vi "Increment.vi"(11 "Data Generator Actor in":refnum<class "Data Generator Actor.lvclass">) -> (3 "Data Generator Actor out":refnum<class "Data Generator Actor.lvclass">)   [LabVIEW 2024, in "Data Generator Actor.lvclass"]
uses:
  Data Generator Actor.lvclass
  Data Generator Actor.lvclass/Data Generator Actor.ctl
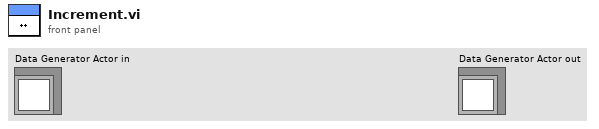
[diagram p1: front panel]
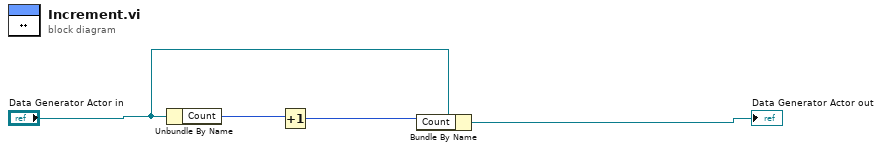
[diagram p0: block diagram]
diagram:
  n1 = Unbundle By Name("Data Generator Actor in") -> ("Count"=w4:i32)
  n2 = Increment(x=w4) -> (x+1=w2:i32)
  n3 = Bundle By Name(cluster="Data Generator Actor in", "Count"=w2) -> (→"Data Generator Actor out":refnum<class "Data Generator Actor.lvclass">)
